vi "Save VI.vi"(6 "Reference Source":T1, 7 "VI Refnum":refnum<vi>, 8 "error in (no error)":errorcluster, 11 "Assert VI Path":path) -> (0 "error out":errorcluster)   [LabVIEW 2018]
uses:
  Save VI Ref Source.ctl
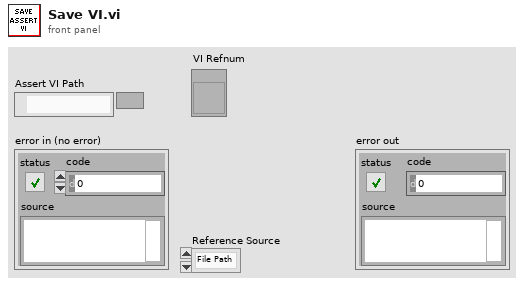
[diagram p1: front panel]
types:
  T1 = typedef "Save VI Ref Source.ctl" = enum16{"File Path", "VI Reference"}
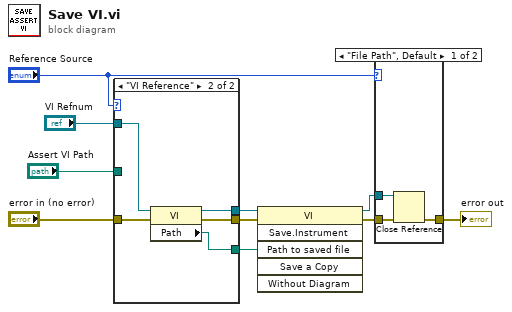
[diagram p0: block diagram]
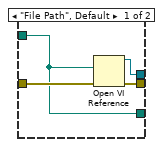
[diagram p3: hidden frame]
diagram:
  n1 = case shown="\"VI Reference\"" "Reference Source" {
    tunnel: "Assert VI Path" -> [w11 _]
    tunnel: [w14 w16] -> w8
    tunnel: [w13 w18] -> w5
    tunnel: "error in (no error)" -> [w12 w19]
    tunnel: "VI Refnum" -> [_ w17]
    tunnel: [w11 w15] -> w1
    frame "File Path", Default {
      n2 = Open VI Reference(vi path=w11, error in (no error)=w12) -> (vi reference=w14:refnum<vi>, error out=w13:errorcluster)  [unwired: 4 in]
    }
    frame "VI Reference" {
      n3 = property class="VI"(reference=w17, error in=w19) -> (reference out=w16:refnum<vi>, error out=w18:errorcluster, "Path"=w15:path)
    }
  }
  n4 = invoke class="VI" method="Save.Instrument"(reference=w8, error in=w5, "Path to saved file"=w1) -> (reference out=w9:refnum<vi>, error out=w6:errorcluster)  [unwired: 3 in, 4 out]
  n5 = case shown="\"File Path\", Default" "Reference Source" {
    tunnel: w9 -> [w22 _]
    tunnel: [w21 w23] -> w7
    tunnel: w6 -> [w20 w23]
    frame "File Path", Default {
      n6 = Close Reference(reference=w22, error in (no error)=w20) -> (error out=w21:errorcluster)
    }
    frame "VI Reference" {
    }
  }
  "error out" <- w7
